vi "Degrees to Arc Length.vi"(5 "Angle":dbl) -> (2 "Arc Length (inches)":dbl)   [LabVIEW 2013]
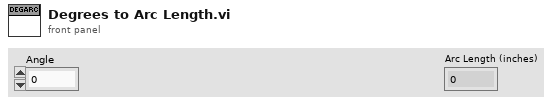
[diagram p1: front panel]
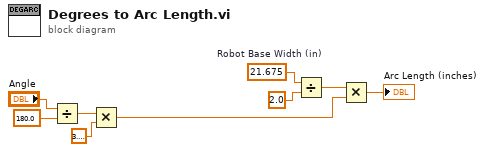
[diagram p0: block diagram]
diagram:
  w8 = 21.675  # Robot Base Width (in)
  n1 = Divide(x="Angle", y=180.0) -> (x/y=w3:dbl)
  n2 = Multiply(x=w3, y=3.141592653589793) -> (x*y=w1:dbl)
  n3 = Divide(x=w8, y=2.0) -> (x/y=w7:dbl)
  n4 = Multiply(x=w7, y=w1) -> (x*y=→"Arc Length (inches)":dbl)
